vi "Compare overlapping.vi"(8 "8":i32, 9 "6":i32, 10 "4":i32, 11 "2":i32) -> (2 "Boolean":bool)   [LabVIEW 2021]
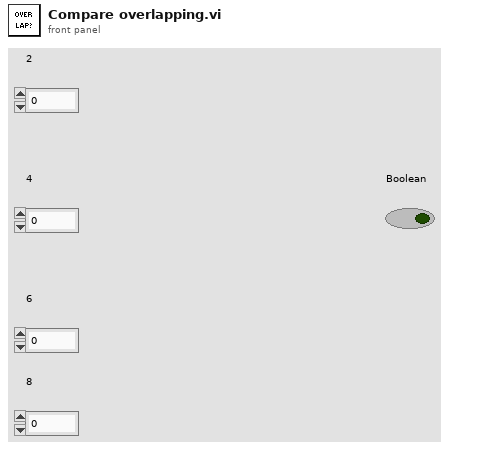
[diagram p1: front panel]
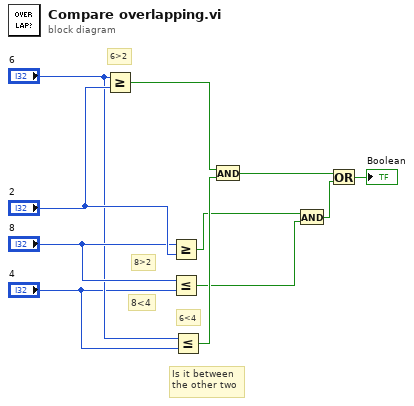
[diagram p0: block diagram]
diagram:
  # "6<4"
  # "8>2"
  # "8<4"
  # "6>2"
  # "Is it between \nthe other two"
  n1 = Greater Or Equal?(x="6", y="2") -> (x >= y?=w7:bool)
  n2 = Greater Or Equal?(x="8", y="2") -> (x >= y?=w1:bool)
  n3 = Less Or Equal?(x="8", y="4") -> (x <= y?=w2:bool)
  n4 = Less Or Equal?(x="6", y="4") -> (x <= y?=w3:bool)
  n5 = And(x=w7, y=w3) -> (x .and. y?=w8:bool)
  n6 = And(x=w1, y=w2) -> (x .and. y?=w9:bool)
  n7 = Or(x=w8, y=w9) -> (x .or. y?=→"Boolean":bool)
